vi "Configure Subframes And Slots.vi"(6 "Meas Subframe (0)":i32, 7 "Subframe Count (1)":i32=1, 8 "error in (no error)":errorcluster, 9 "Subframe Offset (0)":i32, 10 "Instance (1)":T1=1, 11 "VISA resource name":refnum<visa-resource-name>) -> (0 "error out":errorcluster, 3 "VISA resource name out":refnum<visa-resource-name>)   [LabVIEW 2020, in "Rohde&Schwarz CMWXP NR FR1 Measurement.lvlib"]
doc: "Configures which subframes and slots are measured.\n\nAttribute:\nRSCMWXPNRFR1M_ATTR_SUBFRAMES_AND_SLOTS\n\nRemote-control command:\nCONFigure:NRSub:MEAS<i>:MEValuation:MSUBframes"
uses:
  <instrlib>/Rohde&Schwarz CMWXP NR FR1 Measurement/Rohde&Schwarz CMWXP NR FR1 Measurement.lvlib
  <instrlib>/Rohde&Schwarz CMWXP NR FR1 Measurement/Private/_Instance.ctl
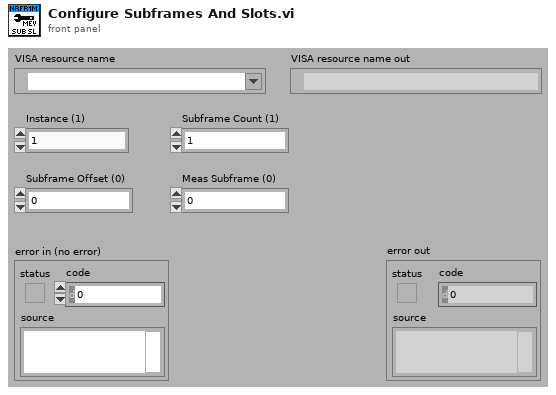
[diagram p1: front panel]
types:
  T1 = typedef "Rohde&Schwarz CMWXP NR FR1 Measurement.lvlib/_Instance.ctl" = i32
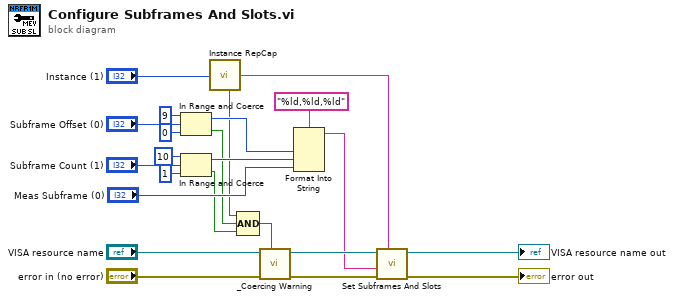
[diagram p0: block diagram]
diagram:
  n1 = In Range and Coerce(upper limit=9, x="Subframe Offset (0)", lower limit=0) -> (coerced(x)=w7:i32, In Range?=w2:bool)
  n2 = In Range and Coerce(upper limit=10, x="Subframe Count (1)", lower limit=1) -> (coerced(x)=w6:i32, In Range?=w3:bool)
  n3 = call <instrlib>:"Instance RepCap.vi"("Instance In"="Instance (1)") -> ("In Range?"=w1:bool, "RepCap Identifier Out"=w20:string)  [unwired: 1 in]
  n4 = Compound Arithmetic op=AND(w1, w2, w3) -> (w9:bool)
  n5 = call <instrlib>:"_Coercing Warning.vi"("In Range?"=w9, "error in (no error)"="error in (no error)", "VISA resource name"="VISA resource name") -> ("error out"=w11:errorcluster, "VISA resource name out"=w10:refnum<visa-resource-name>)  [unwired: 7 in]
  n6 = Format Into String(format string="%ld,%ld,%ld", w7, w6, "Meas Subframe (0)") -> (resulting string=w4:string)  [unwired: 2 in, 1 out]
  n7 = call "Set Subframes And Slots"("Repeated Capabilities"=w20, "error in (no error)"=w11, "Subframes And Slots ()"=w4, "instrument handle"=w10) -> ("error out"=→"error out":errorcluster, "instrument handle out"=→"VISA resource name out":refnum<visa-resource-name>)  [unwired: 6 in]
